vi "LSX Set Trigger Par.vi"(6 "dDistance":dbl, 7 "lSignal":i32, 8 "error in (no error)":errorcluster, 9 "lMode":i32, 10 "lAxis":i32, 11 "lLSID":i32) -> (0 "error out":errorcluster, 3 "function return":i32)   [LabVIEW 2018, in "Tango.lvlib"]
doc: "TANGOAPI int TANGOCALL LSX_SetTriggerPar (int lLSID, int lAxis, int lMode, int lSignal, double dDistance);"
uses:
  <userlib>/Tango/Tango.lvlib
  <userlib>/Tango/Tango_DLL.dll
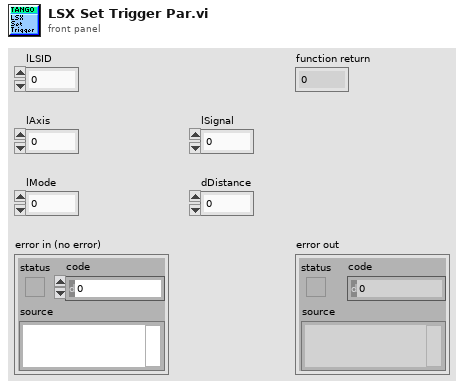
[diagram p1: front panel]
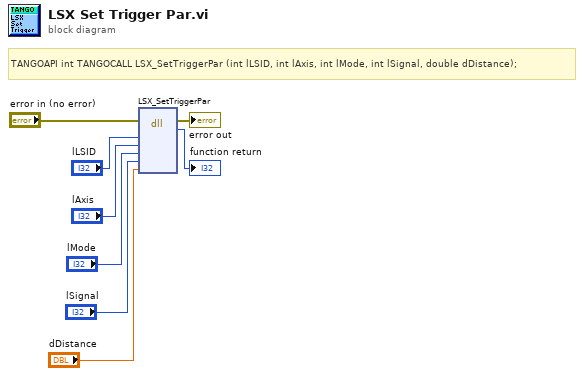
[diagram p0: block diagram]
diagram:
  # "TANGOAPI int TANGOCALL LSX_SetTriggerPar (int lLSID, int lAxis, int lMode, int lSignal, double dDistance);"
  n1 = dll-call lib="C:/Program Files (x86)/National Instruments/LabVIEW 2018/user.lib/Tango/Tango_DLL.*" fn="LSX_SetTriggerPar"(error in="error in (no error)", "lLSID"="lLSID", "lAxis"="lAxis", "lMode"="lMode", "lSignal"="lSignal", "dDistance"="dDistance") -> (error out=→"error out":errorcluster, →"function return":i32)  [unwired: 7 in, 1 out]
